vi "obj tack.vi"() -> ()   [LabVIEW 2019]
uses:
  <vilib>/userDefined/High Color/IMAQdx.ctl
  <vilib>/vision/driver/NI_Vision_Acquisition_Software.lvlib
panel:
  out "Image":T1(plugin-control)
  in  "stop":bool
  out "Image 2":T1(plugin-control)
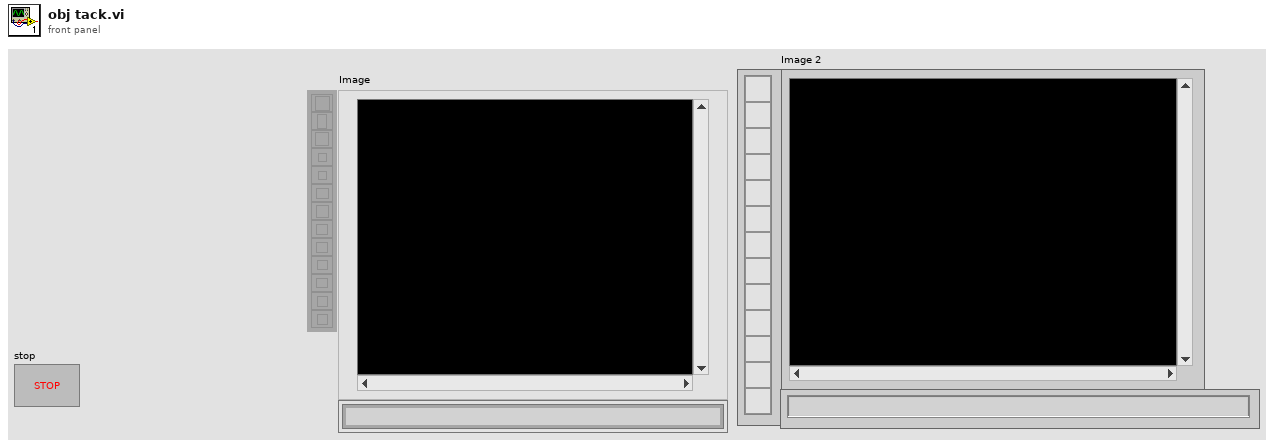
[diagram p1: front panel]
types:
  T1 = typedef "IMAQ Image.ctl" = refnum<image>
  T2 = typedef "IMAQdx.ctl" = refnum<k21>
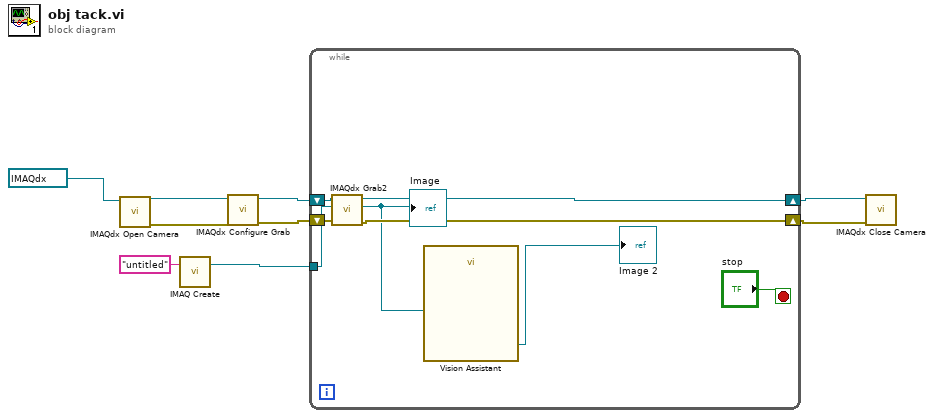
[diagram p0: block diagram]
diagram:
  n1 = call <vilib>:"IMAQdx Open Camera.vi"("Session In"=T2 "cam1") -> ("error out"=w5:errorcluster, "Session Out"=w8:T2)  [unwired: 9 in]
  n2 = call "IMAQ Create"("Image Name"="untitled") -> ("New Image"=w1:T1)  [unwired: 4 in, 1 out]
  n3 = call <vilib>:"IMAQdx Configure Grab.vi"("error in"=w5, "Session In"=w8) -> ("error out"=w4:errorcluster, "Session Out"=w7:T2)  [unwired: 8 in]
  n4 = while {
    tunnel: w1 -> [w13]
    shift-right: [w16] -> w6
    shift-left: w7 -> [w17]
    shift-right: [w14] -> w3
    shift-left: w4 -> [w15]
    stop <- "stop" stop-if-true
    n5 = call <vilib>:"IMAQdx Grab2.vi"("error in"=w15, "Image In"=w13, "Session In"=w17) -> ("error out"=w14:errorcluster, "Image Out"=w10:T1, "Session Out"=w16:T2)  [unwired: 5 in, 1 out]
    "Image" <- w10
    n6 = call "Vision Assistant"("Image In"=w10) -> ("Image Out"=→"Image 2":T1)  [unwired: 25 in, 1 out]
  }
  n7 = call <vilib>:"IMAQdx Close Camera.vi"("error in"=w3, "Session In"=w6) -> ()  [unwired: 9 in, 1 out]
